vi "Browser Workflow Authentication.vi"(4 "Callback Response Body":string="<html>\n<head> <title>Service Verification Tokens Received</title></head>\n<body>\nLabVIEW has received your verification request to use the service. Please close this browser tab and return to the client application to continue using the program!\n</body>\n</html>", 5 "Version (1.0)":string="1.0", 6 "User Login Timeout (120000 ms)":i32=120000, 7 "Signature Method (HMAC-SHA1)":T3=enum."HMAC-SHA1", 8 "error in (no error)":errorcluster, 10 "Authorization URLs":T1, 11 "Client Credentials":T2) -> (0 "error out":errorcluster, 1 "Access Response Body":string, 2 "Access Response Header":string, 3 "OAuth Handle":T4={"Signature Method"=enum."HMAC-SHA1", "Version"="", "Client"={"Token"="", "Secret"=""}, "Access"={"Token"="", "Secret"=""}})   [LabVIEW 2011, in "i3-oauth.lvlib"]
doc: "Uses the <b>Client Credentials</b> that represent this application and the <b>Authorization URLs</b> of the service to receive the Access Credentials for the user's account and create the <b>OAuth Handle</b>.\n\n<b>Additional Information:</b>\nThis VI opens the web browser of the user and directs them to a page where they can log-in and grant permission. This workflow also starts a service on an available TCP port that receives the credentials from the service once the user grants permission. Finally, an OAuth handle is created that includes the Access Credentials for use with the Authenticate with Access Token VI to make requests to the service on behalf of the user.\n\nFor embedded platforms that do not have web browsers or interactive interfaces, the Build OAuth Handle VI can be used to create a handle assuming that Access Credentials have been received through some other method. See Example programs for an example compatible with embedded platforms.\n\n<b>Advanced Information:</b>\nIt is possible to configure the <b>User Login Timeout</b> which is the amout of time the user has available for the web browser to launch, to login to the service, and to grant permissions to this application. After the user grants permission the browser is redirected to a local TCP port hosted by the VI that shows the <b>Callback Response Body</b> as an HTML page. Finally, it is possible to configure the <b>Signature Method</b> to use either HMAC-SHA1 or HMAC-MD5 as specified by the service and the version (which should stay the default of \"1.0\" for OAuth 1.0 and OAuth 1.0a services)."
uses:
  i3-oauth.lvlib
  Controls/OAuth Handle.ctl
  Controls/Signature Method.ctl
  Controls/Credentials.ctl
  Controls/Authorization URLs.ctl
  <vilib>/Platform/browser.llb/Open URL in Default Browser (string).vi
panel:
  out "listening port":u16
  out "remote port":u16
  out "Post Data Transmitted":string
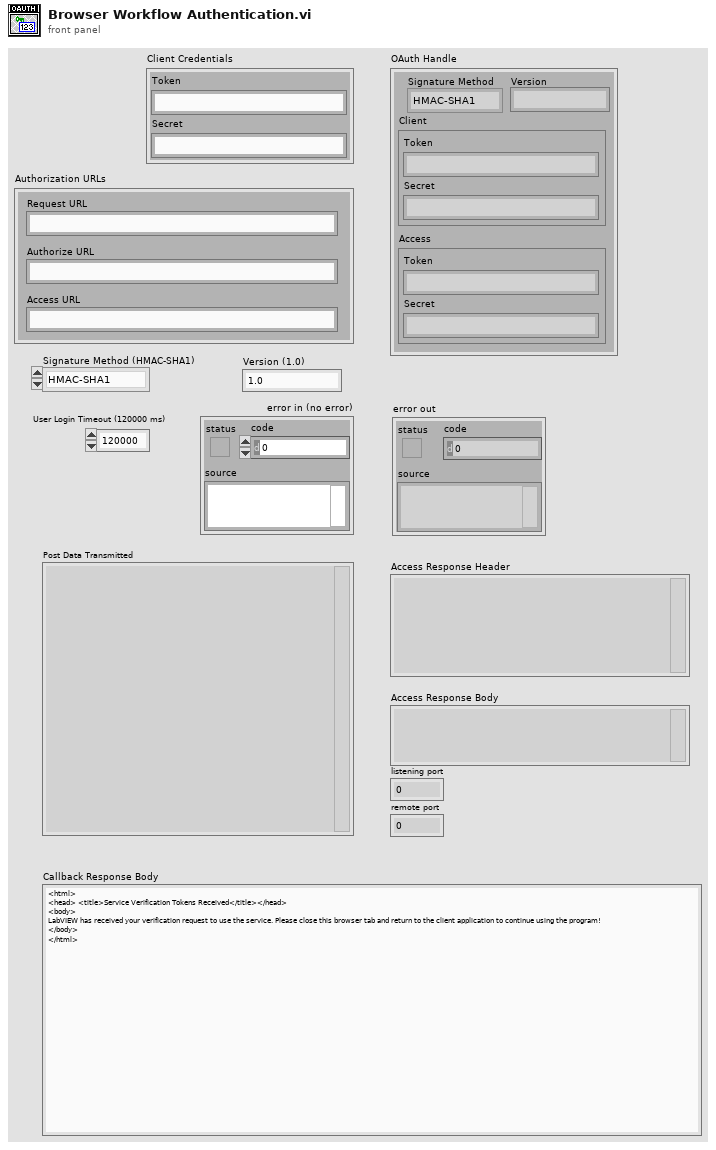
[diagram p1: front panel]
types:
  T1 = typedef "i3-oauth.lvlib/Authorization URLs.ctl" = cluster{"Request URL":string, "Authorize URL":string, "Access URL":string}
  T2 = typedef "i3-oauth.lvlib/Credentials.ctl" = cluster{"Token":string, "Secret":string}
  T3 = typedef "i3-oauth.lvlib/Signature Method.ctl" = enum16{"HMAC-MD5", "HMAC-SHA1", "HMAC-SHA224", "HMAC-SHA256", "HMAC-SHA384", "HMAC-SHA512"}
  T4 = typedef "i3-oauth.lvlib/OAuth Handle.ctl" = cluster{"Signature Method":T3, "Version":string, "Client":T2, "Access":T2}
  T5 = enum16{"Standard", "Buffered", "CRLF", "Immediate"}
  T6 = typedef "i3-oauth.lvlib/Name-Value Pair.ctl" = cluster{"Name":string, "Value":string}
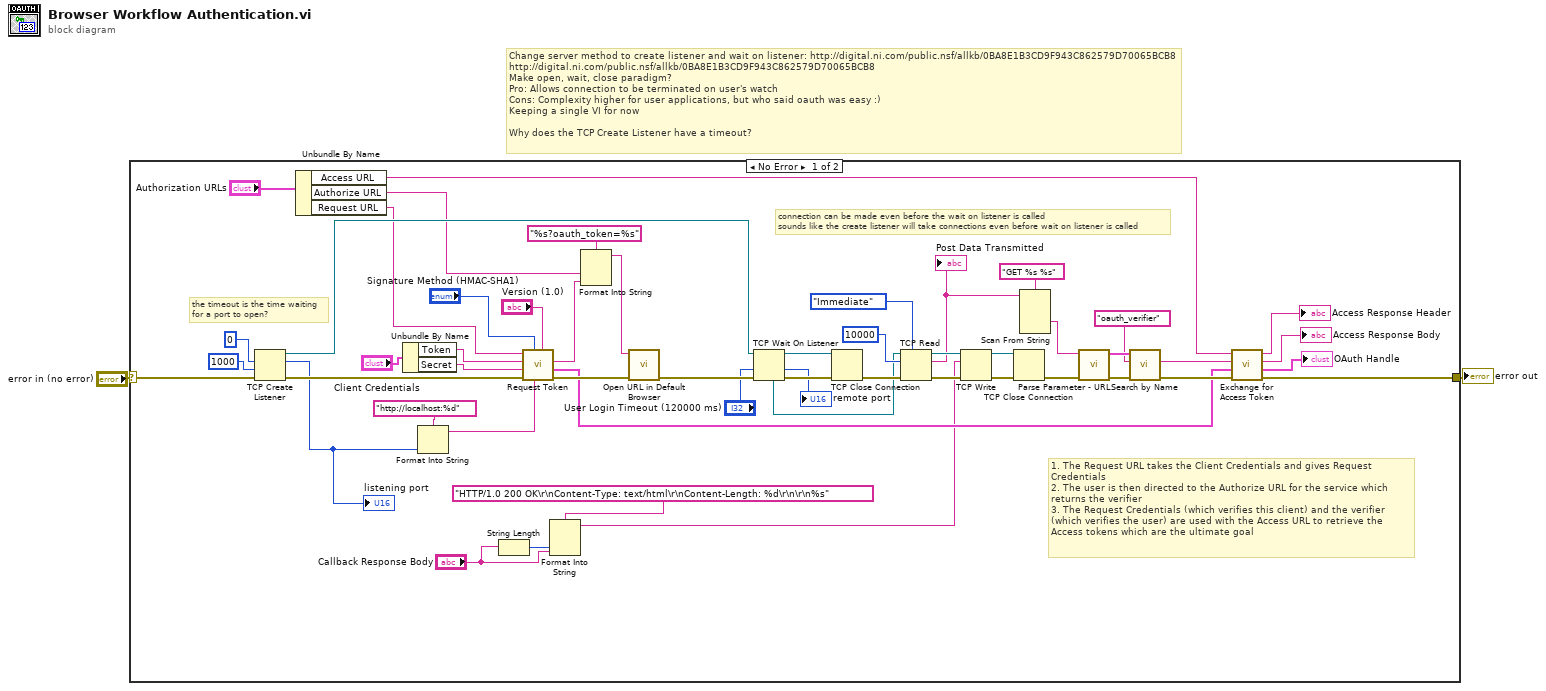
[diagram p0: block diagram]
diagram:
  # "Change server method to create listener and wait on listener: http://digital.ni.com/public.nsf/allkb/0BA8E1B3CD9F943C862579D70065BCB8\nhttp://digital.ni.com/public.nsf/allkb/0BA8E1B3CD9F943C862579D70065BCB8\nMake open, wait, close paradigm?\nPro: Allows connection to be terminated on user's watch\nCons: Complexity higher for user applications, but who said oauth was easy :)\nKeeping a single VI for now\n\nWhy does the TCP Create Listener have a timeout?"
  n1 = case shown="No Error" "error in (no error)" {
    selector: "error in (no error)" -> [w21 w55]
    tunnel: [w48 w55] -> w1
    frame No Error {
      # "1. The Request URL takes the Client Credentials and gives Request Credentials\n2. The user is then directed to the Authorize URL for the service which returns the verifier\n3. The Request Credentials (which verifies this client) and the verifier (which verifies the user) are used with the Access URL to retrieve the Access tokens which are the ultimate goal"
      # "the timeout is the time waiting \nfor a port to open?"
      # "connection can be made even before the wait on listener is called\nsounds like the create listener will take connections even before wait on listener is called"
      n2 = TCP Create Listener(8:w21, 9:1000 ("timeout ms (25000)"), 10:u16 0 ("port")) -> (0:w22:errorcluster, 2:w18:u16, 3:w17:refnum<k5>)  [unwired: 2 in]
      "listening port" <- w18
      n3 = Unbundle By Name("Authorization URLs") -> ("Access URL"=w3:string, "Authorize URL"=w4:string, "Request URL"=w5:string)
      n4 = Unbundle By Name("Client Credentials") -> ("Token"=w9:string, "Secret"=w8:string)
      n5 = Format Into String(format string="http://localhost:%d" ("string"), w18) -> (resulting string=w44:string)  [unwired: 2 in, 1 out]
      n6 = String Length(string="Callback Response Body") -> (length=w25:i32)
      n7 = call "Request Token.vi"("Version"="Version (1.0)", "Callback URL"=w44, "Signature Method"="Signature Method (HMAC-SHA1)", "error in (no error)"=w22, "Consumer Secret"=w8, "Consumer Key"=w9, "Request URL"=w5) -> ("error out"=w53:errorcluster, "OAuth Credentials (request)"=w50:T4, "Request Token (duplicate)"=w37:string)  [unwired: 2 in]
      n8 = Format Into String(format string="HTTP/1.0 200 OK\r\nContent-Type: text/html\r\nContent-Length: %d\r\n\r\n%s" ("data in"), w25, "Callback Response Body") -> (resulting string=w23:string)  [unwired: 2 in, 1 out]
      n9 = Format Into String(format string="%s?oauth_token=%s", w4, w37) -> (resulting string=w35:string)  [unwired: 2 in, 1 out]
      n10 = call-poly <vilib>:"Open URL in Default Browser.vi"("error in (no error)"=w53, "URL"=w35) -> ("error out"=w54:errorcluster)  [unwired: 4 in, 1 out]
      n11 = TCP Wait On Listener(8:w54, 9:"User Login Timeout (120000 ms)", 11:w17) -> (0:w15:errorcluster, 1:→"remote port":u16, 3:w13:refnum<k5>, 4:w12:refnum<k5>)  [unwired: 1 in, 1 out]
      n12 = TCP Close Connection(connection ID=w13, error in (no error)=w15) -> (error out=w14:errorcluster)  [unwired: 1 in, 1 out]
      n13 = TCP Read(connection ID=w12, bytes to read=10000, error in (no error)=w14, 7:T5."Immediate" ("mode (standard)")) -> (connection ID out=w42:refnum<k5>, data out=w31:string, error out=w41:errorcluster)  [unwired: 1 in]
      "Post Data Transmitted" <- w31
      n14 = TCP Write(connection ID=w42, data in=w23, error in (no error)=w41) -> (connection ID out=w39:refnum<k5>, error out=w40:errorcluster)  [unwired: 1 in, 1 out]
      n15 = TCP Close Connection(connection ID=w39, error in (no error)=w40) -> (error out=w34:errorcluster)  [unwired: 1 in, 1 out]
      n16 = Scan From String(format string="GET %s %s", input string=w31) -> (output 1=w30:string)  [unwired: 5 in, 3 out]
      n17 = call "Parse Parameter - URL.vi"("error in (no error)"=w34, "URL"=w30) -> ("error out"=w33:errorcluster, "URL Parameters"=w29:T6[])  [unwired: 8 in]
      n18 = call "Search by Name.vi"("error in (no error)"=w33, "Name"="oauth_verifier" ("Key"), "Name-Value Pair List"=w29) -> ("error out"=w52:errorcluster, "Value"=w27:string)  [unwired: 6 in, 1 out]
      n19 = call "Exchange for Access Token.vi"("error in (no error)"=w52, "OAuth Credentials (request)"=w50, "Pin"=w27, "Access Request URL"=w3) -> ("error out"=w48:errorcluster, "OAuth Credentials (access)"=→"OAuth Handle":T4, "body"=→"Access Response Body":string, "headers"=→"Access Response Header":string)  [unwired: 4 in]
    }
    frame Error {
    }
  }
  "error out" <- w1
